vi "Plot default properties.vi"() -> (0 "General":T1={"Title"="Title", "Time to Plot"=1800.0, "Title.Visible"=TRUE, "Sidebar.Visible"=FALSE, "Plot Area:Colors:BG Color"=0, "X Scale.Plot Name"="", "X Scale.Use Plot Name"=FALSE} {"Time to Plot" format="%<%M:%S>t"}, 1 "Default Y-axes":T3[](array[typedef])=[{"Name Label.Text"="Left Axis", "Style"=0, "Tick Colors:Minor Tick Color"=16777216, "Tick Colors:Tick Color"=3684408, "Marker Colors:Text Color"=16448250, "Grid Colors:Major Color"=3684408, "Grid Colors:Minor Color"=16777216, "Mapping Mode"=0, "Flipped"=FALSE, "Name Label.Visible"=FALSE, "Name Label.Text Colors:Text Color"=16448250, "Scale Fit"=2, "Range:Maximum"=1.0, "Range:Minimum"=0.0, "Offset and Multiplier:Multiplier"=1.0, "Offset and Multiplier:Offset"=0.0, "Name Label.Font:Size"=15, "Marker.Font:Size"=15, "Uniform Marker Spacing?"=TRUE, "Format String"="%#_g"}, {"Name Label.Text"="Right Axis", "Style"=0, "Tick Colors:Minor Tick Color"=16777216, "Tick Colors:Tick Color"=3684408, "Marker Colors:Text Color"=16448250, "Grid Colors:Major Color"=3684408, "Grid Colors:Minor Color"=16777216, "Mapping Mode"=0, "Flipped"=FALSE, "Name Label.Visible"=FALSE, "Name Label.Text Colors:Text Color"=16448250, "Scale Fit"=2, "Range:Maximum"=1.0, "Range:Minimum"=0.0, "Offset and Multiplier:Multiplier"=1.0, "Offset and Multiplier:Offset"=0.0, "Name Label.Font:Size"=15, "Marker.Font:Size"=15, "Uniform Marker Spacing?"=TRUE, "Format String"="%#_g"}], 2 "Default X-axis":T3={"Name Label.Text"="Time (s)", "Style"=0, "Tick Colors:Minor Tick Color"=16777216, "Tick Colors:Tick Color"=3684408, "Marker Colors:Text Color"=16448250, "Grid Colors:Major Color"=3684408, "Grid Colors:Minor Color"=16777216, "Mapping Mode"=0, "Flipped"=FALSE, "Name Label.Visible"=FALSE, "Name Label.Text Colors:Text Color"=16448250, "Scale Fit"=2, "Range:Maximum"=3530119305.0, "Range:Minimum"=3530119285.0, "Offset and Multiplier:Multiplier"=1.0, "Offset and Multiplier:Offset"=0.0, "Name Label.Font:Size"=15, "Marker.Font:Size"=15, "Uniform Marker Spacing?"=TRUE, "Format String"="%<%H:%M:%S>T"}, 3 "Default Attributes":T4={"Plot Color"=16711680, "Point Style"=0, "Line Style"=0, "Plot Interpolation"=2, "Line Width"=0, "Bar Plot Style"=0, "Fill To"=-1, "X Scale Index"=0, "Y Scale Index"=0, "Anti-aliased"=FALSE, "Label Format"=3, "Digital Transition Type"=0, "Digital Transition Location"=2, "Digital Line Style"=1, "Fill/Point Color"=16777215, "Plot Name"="", "Visible"=TRUE}, 4 "Default plot UI":T2={"PID"="", "index"=0, "PID color"=16777225, "right axis?"=FALSE, "Flatline?"=FALSE, "Numeric color"=0, "Data"="", "Flat"=""})   [LabVIEW 2021, in "RocketPlot.lvlib"]
uses:
  RocketPlot.lvlib
  TypeDefs/plot attributes V2.ctl
  TypeDefs/Plot scale axis properties.ctl
  TypeDefs/Plot top row.ctl
  TypeDefs/Plot general properties.ctl
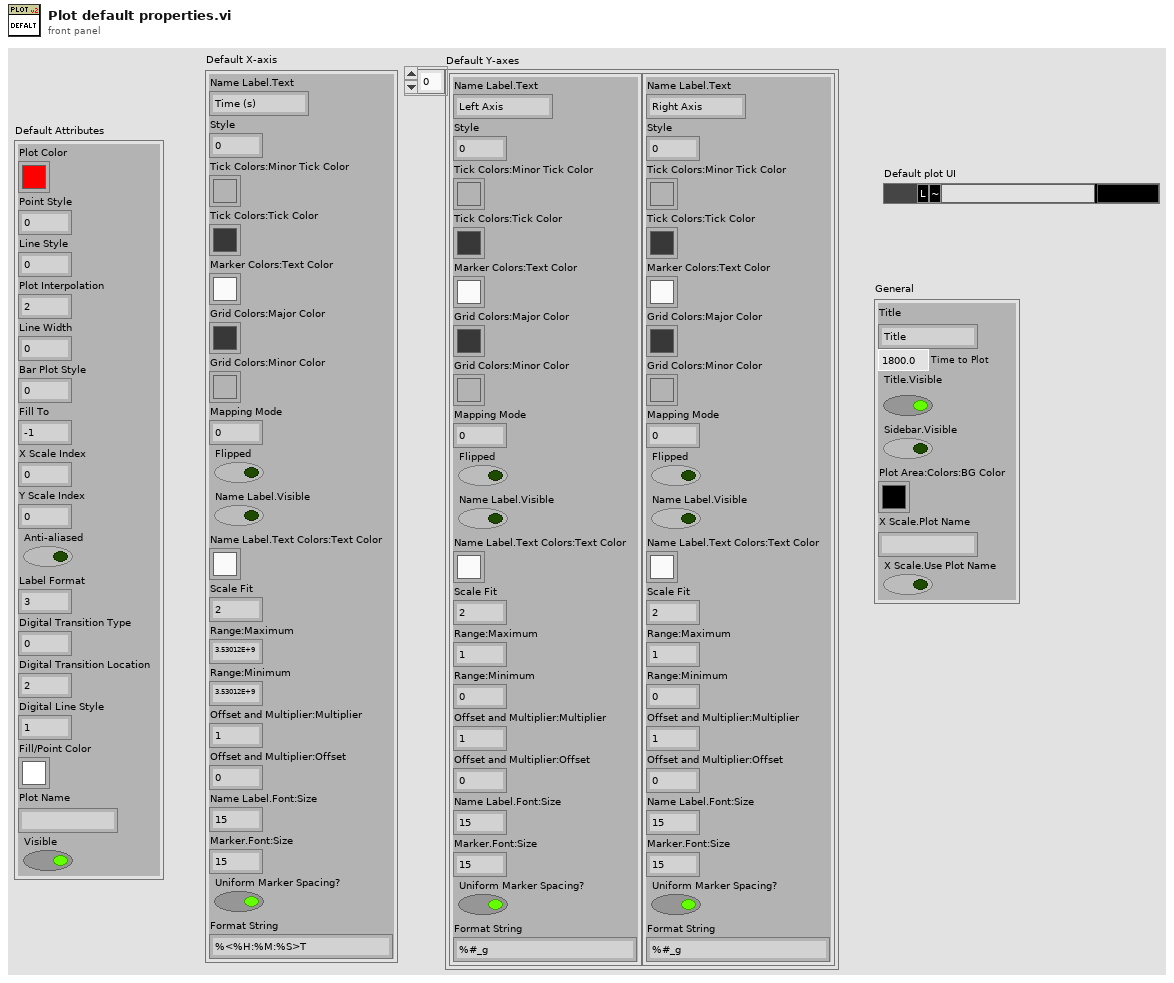
[diagram p1: front panel]
types:
  T1 = typedef "RocketPlot.lvlib/Plot general properties.ctl" = cluster{"Title":string, "Time to Plot":dbl, "Title.Visible":bool, "Sidebar.Visible":bool, "Plot Area:Colors:BG Color":u32, "X Scale.Plot Name":string, "X Scale.Use Plot Name":bool}
  T2 = typedef "RocketPlot.lvlib/Plot top row.ctl" = cluster{"PID":string, "index":i32, "PID color":u32, "right axis?":bool, "Flatline?":bool, "Numeric color":u32, "Data":string, "Flat":string}
  T3 = typedef "RocketPlot.lvlib/Plot scale axis properties.ctl" = cluster{"Name Label.Text":string, "Style":u8, "Tick Colors:Minor Tick Color":u32, "Tick Colors:Tick Color":u32, "Marker Colors:Text Color":u32, "Grid Colors:Major Color":u32, "Grid Colors:Minor Color":u32, "Mapping Mode":u8, "Flipped":bool, "Name Label.Visible":bool, "Name Label.Text Colors:Text Color":u32, "Scale Fit":u8, "Range:Maximum":dbl, "Range:Minimum":dbl, "Offset and Multiplier:Multiplier":dbl, "Offset and Multiplier:Offset":dbl, "Name Label.Font:Size":u32, "Marker.Font:Size":u32, "Uniform Marker Spacing?":bool, "Format String":string}
  T4 = typedef "RocketPlot.lvlib/plot attributes V2.ctl" = cluster{"Plot Color":u32, "Point Style":u8, "Line Style":u8, "Plot Interpolation":u8, "Line Width":u8, "Bar Plot Style":u8, "Fill To":i16, "X Scale Index":u32, "Y Scale Index":u32, "Anti-aliased":bool, "Label Format":u8, "Digital Transition Type":u8, "Digital Transition Location":u8, "Digital Line Style":u8, "Fill/Point Color":u32, "Plot Name":string, "Visible":bool}
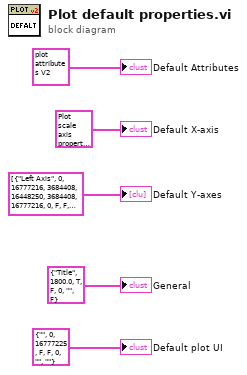
[diagram p0: block diagram]
diagram:
  "Default Attributes" <- T4 {"Plot Color"=16711680, "Point Style"=0, "Line Style"=0, "Plot Interpolation"=2, "Line Width"=0, "Bar Plot Style"=0, "Fill To"=-1, "X Scale Index"=0, "Y Scale Index"=0, "Anti-aliased"=FALSE, "Label Format"=3, "Digital Transition Type"=0, "Digital Transition Location"=2, "Digital Line Style"=1, "Fill/Point Color"=16777215, "Plot Name"="", "Visible"=TRUE} ("Default Attributes")
  "Default X-axis" <- T3 {"Name Label.Text"="Time (s)", "Style"=0, "Tick Colors:Minor Tick Color"=16777216, "Tick Colors:Tick Color"=3684408, "Marker Colors:Text Color"=16448250, "Grid Colors:Major Color"=3684408, "Grid Colors:Minor Color"=16777216, "Mapping Mode"=0, "Flipped"=FALSE, "Name Label.Visible"=FALSE, "Name Label.Text Colors:Text Color"=16448250, "Scale Fit"=2, "Range:Maximum"=3530119305.0, "Range:Minimum"=3530119285.0, "Offset and Multiplier:Multiplier"=1.0, "Offset and Multiplier:Offset"=0.0, "Name Label.Font:Size"=15, "Marker.Font:Size"=15, "Uniform Marker Spacing?"=TRUE, "Format String"="%<%H:%M:%S>T"} ("Default X-axis")
  "Default Y-axes" <- T3[] [{"Name Label.Text"="Left Axis", "Style"=0, "Tick Colors:Minor Tick Color"=16777216, "Tick Colors:Tick Color"=3684408, "Marker Colors:Text Color"=16448250, "Grid Colors:Major Color"=3684408, "Grid Colors:Minor Color"=16777216, "Mapping Mode"=0, "Flipped"=FALSE, "Name Label.Visible"=FALSE, "Name Label.Text Colors:Text Color"=16448250, "Scale Fit"=2, "Range:Maximum"=1.0, "Range:Minimum"=0.0, "Offset and Multiplier:Multiplier"=1.0, "Offset and Multiplier:Offset"=0.0, "Name Label.Font:Size"=15, "Marker.Font:Size"=15, "Uniform Marker Spacing?"=TRUE, "Format String"="%#_g"}, {"Name Label.Text"="Right Axis", "Style"=0, "Tick Colors:Minor Tick Color"=16777216, "Tick Colors:Tick Color"=3684408, "Marker Colors:Text Color"=16448250, "Grid Colors:Major Color"=3684408, "Grid Colors:Minor Color"=16777216, "Mapping Mode"=0, "Flipped"=FALSE, "Name Label.Visible"=FALSE, "Name Label.Text Colors:Text Color"=16448250, "Scale Fit"=2, "Range:Maximum"=1.0, "Range:Minimum"=0.0, "Offset and Multiplier:Multiplier"=1.0, "Offset and Multiplier:Offset"=0.0, "Name Label.Font:Size"=15, "Marker.Font:Size"=15, "Uniform Marker Spacing?"=TRUE, "Format String"="%#_g"}] ("Default Y-axes")
  "Default plot UI" <- T2 {"PID"="", "index"=0, "PID color"=16777225, "right axis?"=FALSE, "Flatline?"=FALSE, "Numeric color"=0, "Data"="", "Flat"=""} ("Default plot UI")
  "General" <- T1 {"Title"="Title", "Time to Plot"=1800.0, "Title.Visible"=TRUE, "Sidebar.Visible"=FALSE, "Plot Area:Colors:BG Color"=0, "X Scale.Plot Name"="", "X Scale.Use Plot Name"=FALSE} ("General")
